vi "Analog Input.vi"(6 "clai. Parmeter":T1, 8 "error in":errorcluster, 9 "Min Value":string[](array[string]), 10 "Max Value":string[](array[string]), 11 "DAQmx Analog Input Setting":T2={"DAQmx Analog Input_00"="Dev1/ai0", "DAQmx Analog Input_01"="Dev1/ai1", "DAQmx Analog Input_02"="Dev1/ai2", "DAQmx Analog Input_03"="Dev1/ai3", "DAQmx Analog Input_04"="Dev1/ai4", "DAQmx Analog Input_05"="Dev1/ai5", "DAQmx Analog Input_06"="Dev1/ai6", "DAQmx Analog Input_07"="Dev1/ai7", "DAQmx Analog Input_00 2"="Dev1/ai8", "DAQmx Analog Input_01 2"="Dev1/ai9", "DAQmx Analog Input_02 2"="Dev1/ai10", "DAQmx Analog Input_03 2"="Dev1/ai11", "DAQmx Analog Input_04 2"="Dev1/ai12", "DAQmx Analog Input_05 2"="Dev1/ai13", "DAQmx Analog Input_06 2"="Dev1/ai14", "DAQmx Analog Input_07 2"="Dev1/ai15", "DAQmx Analog Input_00 3"="Dev1/ai16", "DAQmx Analog Input_01 3"="Dev1/ai17", "DAQmx Analog Input_02 3"="Dev1/ai18", "DAQmx Analog Input_03 3"="Dev1/ai19", "DAQmx Analog Input_04 3"="Dev1/ai20", "DAQmx Analog Input_05 3"="Dev1/ai21", "DAQmx Analog Input_06 3"="Dev1/ai22", "DAQmx Analog Input_07 3"="Dev1/ai23", "DAQmx Analog Input_00 4"="Dev1/ai24", "DAQmx Analog Input_01 4"="Dev1/ai25", "DAQmx Analog Input_02 4"="Dev1/ai26", "DAQmx Analog Input_03 4"="Dev1/ai27", "DAQmx Analog Input_04 4"="Dev1/ai28", "DAQmx Analog Input_05 4"="Dev1/ai29", "DAQmx Analog Input_06 4"="Dev1/ai30", "DAQmx Analog Input_07 4"="Dev1/ai31"}) -> (0 "error out":errorcluster, 1 "Exit":bool)   [LabVIEW 2015]
uses:
  <vilib>/DAQmx/read.llb/DAQmx Read (Analog 2D DBL NChan NSamp).vi
  <vilib>/DAQmx/create/channels.llb/DAQmx Create Channel (AI-Voltage-Basic).vi
  <vilib>/DAQmx/configure/timing.llb/DAQmx Timing (Sample Clock).vi
  Galobal variable_TI.vi
  <vilib>/DAQmx/miscellaneous.llb/DAQmx Fill In Error Info.vi
panel:
  out "Boolean":bool
  out "Waveform Chart":dbl(graph)
  out "element":dbl
  out "x-y":u32
  out "error out 2":errorcluster
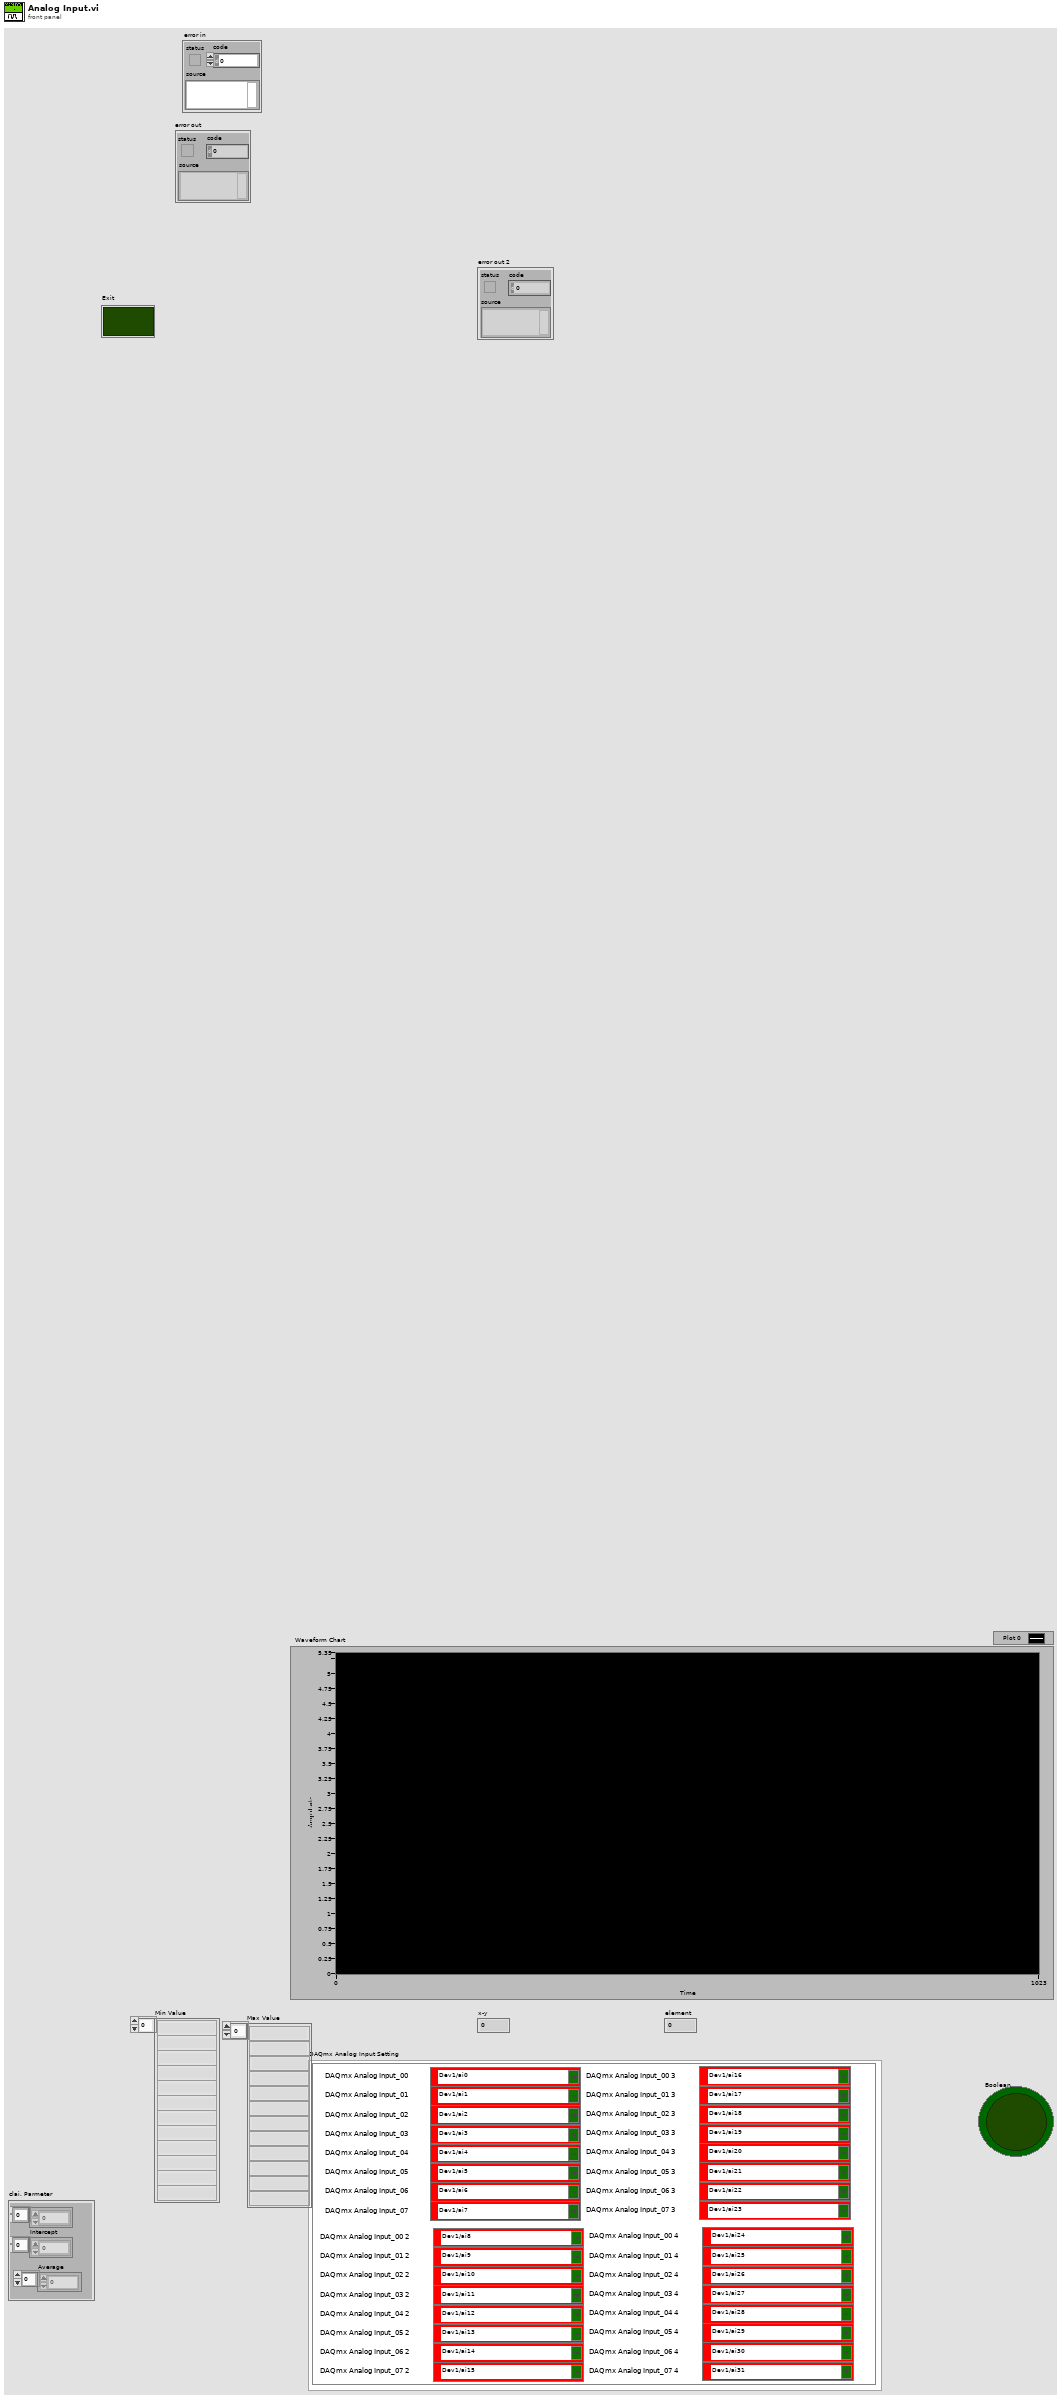
[diagram p1: front panel]
types:
  T1 = cluster{"Slop":dbl[], "Intercept":dbl[], "Average ":i16[]}
  T2 = cluster{"DAQmx Analog Input_00":tag, "DAQmx Analog Input_01":tag, "DAQmx Analog Input_02":tag, "DAQmx Analog Input_03":tag, "DAQmx Analog Input_04":tag, "DAQmx Analog Input_05":tag, "DAQmx Analog Input_06":tag, "DAQmx Analog Input_07":tag, "DAQmx Analog Input_00 2":tag, "DAQmx Analog Input_01 2":tag, "DAQmx Analog Input_02 2":tag, "DAQmx Analog Input_03 2":tag, "DAQmx Analog Input_04 2":tag, "DAQmx Analog Input_05 2":tag, "DAQmx Analog Input_06 2":tag, "DAQmx Analog Input_07 2":tag, "DAQmx Analog Input_00 3":tag, "DAQmx Analog Input_01 3":tag, "DAQmx Analog Input_02 3":tag, "DAQmx Analog Input_03 3":tag, "DAQmx Analog Input_04 3":tag, "DAQmx Analog Input_05 3":tag, "DAQmx Analog Input_06 3":tag, "DAQmx Analog Input_07 3":tag, "DAQmx Analog Input_00 4":tag, "DAQmx Analog Input_01 4":tag, "DAQmx Analog Input_02 4":tag, "DAQmx Analog Input_03 4":tag, "DAQmx Analog Input_04 4":tag, "DAQmx Analog Input_05 4":tag, "DAQmx Analog Input_06 4":tag, "DAQmx Analog Input_07 4":tag}
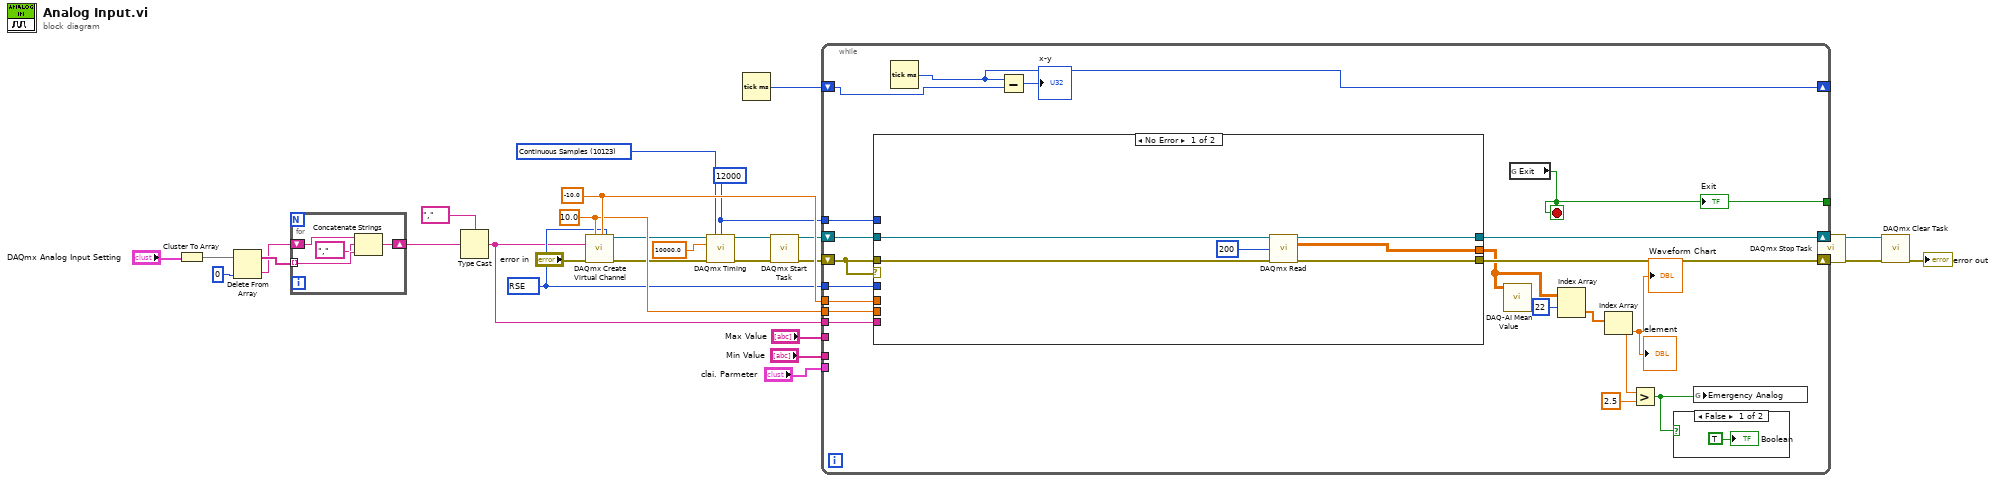
[diagram p0: block diagram]
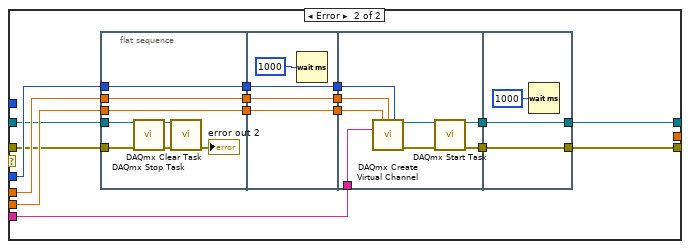
[diagram p3: hidden frame]
diagram:
  w8 = 12000 ("samples per channel")
  w23 = 10123 items=["Finite Samples"=10178, "Continuous Samples"=10123, "Hardware Timed Single Point"=12522] ("sample mode")
  w29 = 10083 items=["default"=-1, "RSE"=10083, "NRSE"=10078, "Differential"=10106, "Pseudodifferential"=12529] ("input terminal configuration")
  w31 = -10.0 ("minimum value")
  w30 = 10.0 ("maximum value")
  n1 = Cluster To Array(cluster="DAQmx Analog Input Setting") -> (array=w20:tag[])
  n2 = Delete From Array(array=w20, index=0) -> (deleted portion=w17:tag, array with subset deleted=w19:tag[])  [unwired: 1 in]
  n3 = for {
    tunnel: w19 -> [w35] mode=indexing
    shift-right: [w33] -> w15
    shift-left: w17 -> [w32]
    n4 = Concatenate Strings(w32, tag "," ("1."), w35) -> (w33:string)
  }
  n5 = Type Cast(type=tag "," ("1."), x=w15) -> (*(type *) &x=w21:tag)
  n6 = call-poly <vilib>:"DAQmx Create Virtual Channel.vi"("maximum value"=w30, "minimum value"=w31, "input terminal configuration"=w29, "physical channels"=w21, "error in"="error in") -> ("task out"=w27:refnum<k21>, "error out"=w26:errorcluster)  [unwired: 4 in, 5 out]
  n7 = call-poly <vilib>:"DAQmx Timing.vi"("task/channels in"=w27, "sample mode"=w23, "samples per channel"=w8, "rate"=10000.0, "error in"=w26) -> ("task out"=w25:refnum<k21>, "error out"=w24:errorcluster)  [unwired: 9 in]
  n8 = Tick Count (ms)() -> (millisecond timer value=w7:u32)
  n9 = call <vilib>:"DAQmx Start Task.vi"("task/channels in"=w25, "error in"=w24) -> ("task out"=w13:refnum<k21>, "error out"=w12:errorcluster)  [unwired: 12 out]
  n10 = while {
    shift-right: [w51] -> w11
    shift-left: w12 -> [w54]
    shift-right: [w52] -> w10
    shift-left: w13 -> [w53]
    tunnel: w21 -> [w50]
    tunnel: w31 -> [w49]
    tunnel: w30 -> [w48]
    tunnel: w29 -> [w47]
    tunnel: [w46] -> w9
    tunnel: w8 -> [w45]
    shift-right: [w43] -> _
    shift-left: w7 -> [w44]
    tunnel: "Max Value" -> [_]
    tunnel: "Min Value" -> [_]
    tunnel: "clai. Parmeter" -> [_]
    stop <- w46 stop-if-true
    n11 = case shown="No Error" w54 {
      tunnel: w54 -> [w60 w64]
      tunnel: w53 -> [w61 w65]
      tunnel: [w59 w63] -> w52
      tunnel: [w58 w62] -> w51
      tunnel: w50 -> [_ w77]
      tunnel: w49 -> [_ w76]
      tunnel: w48 -> [_ w75]
      tunnel: w47 -> [_ w74]
      tunnel: [w57 _] -> w41
      tunnel: w45 -> [_ _]
      frame No Error {
        n12 = call-poly <vilib>:"DAQmx Read.vi"("task/channels in"=w61, "number of samples per channel"=200, "error in"=w60) -> ("task out"=w59:refnum<k21>, "data"=w57:dbl[][], "error out"=w58:errorcluster)  [unwired: 10 out]
      }
      frame Error {
        n13 = flat-sequence {
          tunnel: w74 -> [w83]
          tunnel: w75 -> [w84]
          tunnel: w76 -> [w85]
          tunnel: [w85] -> w68
          tunnel: [w84] -> w67
          tunnel: [w83] -> w66
          tunnel: w65 -> [w81]
          tunnel: w64 -> [w80]
          tunnel: [w89] -> w71
          tunnel: [w88] -> w70
          tunnel: [w87] -> w69
          tunnel: w68 -> [w89]
          tunnel: w67 -> [w88]
          tunnel: w66 -> [w87]
          tunnel: w77 -> [w95]
          tunnel: [w91] -> w73
          tunnel: [w90] -> w72
          tunnel: w71 -> [w94]
          tunnel: w70 -> [w93]
          tunnel: w69 -> [w92]
          tunnel: [w99] -> w62
          tunnel: [w100] -> w63
          tunnel: w73 -> [w100]
          tunnel: w72 -> [w99]
          frame #0 {
            n14 = call <vilib>:"DAQmx Stop Task.vi"("task/channels in"=w81, "error in"=w80) -> ("task out"=w78:refnum<k21>, "error out"=w82:errorcluster)  [unwired: 12 in]
            n15 = call <vilib>:"DAQmx Clear Task.vi"("task in"=w78, "error in"=w82) -> ("error out"=→"error out 2":errorcluster)  [unwired: 13 in]
          }
          frame #1 {
            n16 = Wait (ms)(milliseconds to wait=u32 1000) -> ()  [unwired: 1 out]
          }
          frame #2 {
            n17 = call-poly <vilib>:"DAQmx Create Virtual Channel.vi"("maximum value"=w93, "minimum value"=w94, "input terminal configuration"=w92, "physical channels"=w95) -> ("task out"=w97:refnum<k21>, "error out"=w96:errorcluster)  [unwired: 5 in, 5 out]
            n18 = call <vilib>:"DAQmx Start Task.vi"("task/channels in"=w97, "error in"=w96) -> ("task out"=w91:refnum<k21>, "error out"=w90:errorcluster)  [unwired: 12 out]
          }
          frame #3 {
            n19 = Wait (ms)(milliseconds to wait=u32 1000) -> ()  [unwired: 1 out]
          }
        }
      }
    }
    n20 = Tick Count (ms)() -> (millisecond timer value=w43:u32)
    n21 = Subtract(x=w43, y=w44) -> (x-y=→"x-y":u32)
    n22 = call "DAQ-AI Mean Value.vi"("data"=w41) -> ()  [unwired: 10 in, 1 out]
    n23 = global read "Galobal variable_TI.vi" "Exit"() -> (w46:bool)
    n24 = Index Array(array=w41, index (row)=22) -> (element=w39:dbl[])  [unwired: 1 in]
    n25 = Index Array(array=w39) -> (element=w38:dbl)  [unwired: 1 in]
    "element" <- w38
    "Waveform Chart" <- w38
    n26 = Greater?(x=w38, y=2.5) -> (0:w36:bool)
    n27 = case shown="False" w36 {
      frame False {
        "Boolean" <- TRUE ("Boolean")
      }
      frame True {
      }
    }
    n28 = global write "Galobal variable_TI.vi" "Emergency Analog"(w36) -> ()
  }
  "Exit" <- w9
  n29 = call <vilib>:"DAQmx Stop Task.vi"("task/channels in"=w10, "error in"=w11) -> ("task out"=w4:refnum<k21>, "error out"=w3:errorcluster)  [unwired: 12 in]
  n30 = call <vilib>:"DAQmx Clear Task.vi"("task in"=w4, "error in"=w3) -> ("error out"=→"error out":errorcluster)  [unwired: 13 in]
